vi "Furnace_VI.vi"() -> ()   [LabVIEW 2014]
uses:
  <vilib>/rvi/Emulation/niFpgaGetClockAttributes.vi
  <vilib>/rvi/Emulation/niFpgaSctlEmulationGetInTimedLoop.vi
  <vilib>/rvi/Emulation/niFpgaEmulationReportErrorSimple.vi
  <vilib>/rvi/Emulation/niFpgaCriticalErrorInLSC.vi
panel:
  out "appended array":u8[](array[numeric])
  in  "Command":i16
  in  "Ramp rate,SP&CRC":u8[](array[numeric])=[66, 0, 0, 0, 132, 246]
  in  "Furnace Array Out":u8[](array[numeric])=[65, 48, 48, 48, 48, 48, 13, 68, 48, 48, 48, 48]
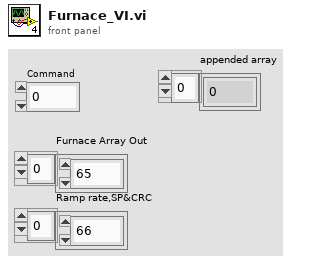
[diagram p1: front panel]
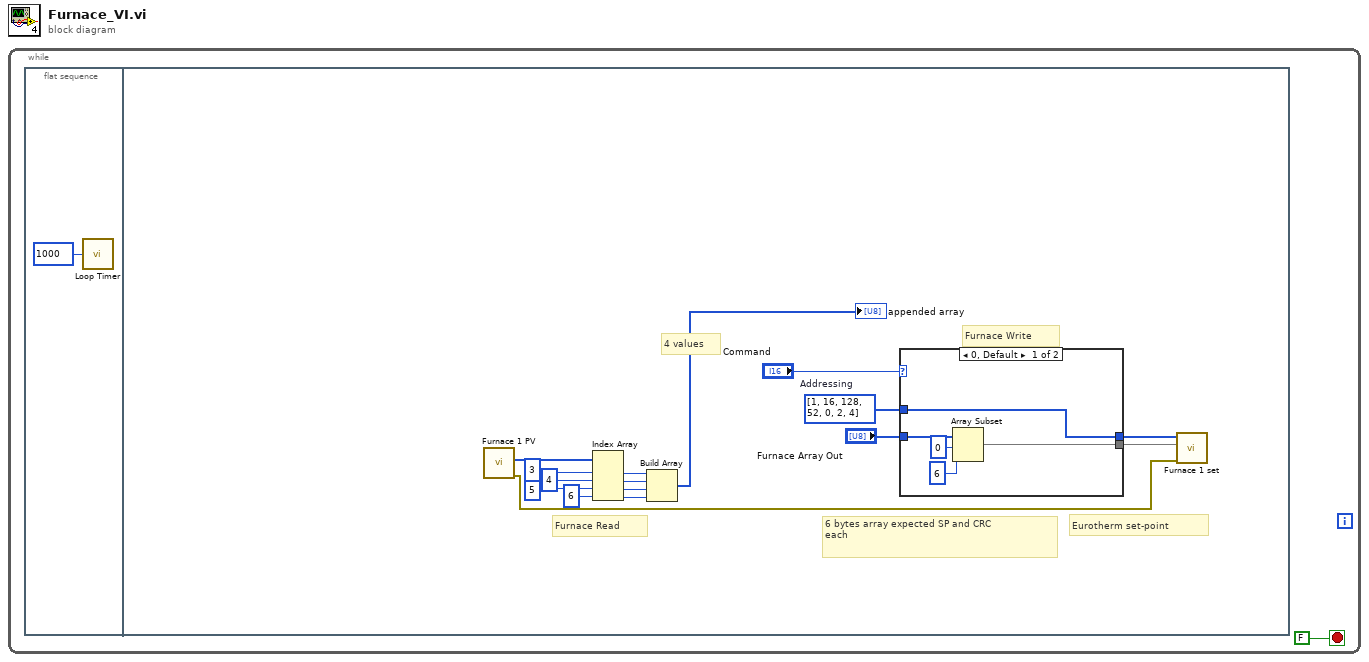
[diagram p0: block diagram]
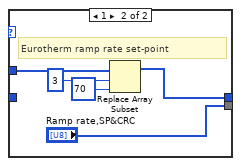
[diagram p2: hidden frame]
diagram:
  n1 = while {
    stop <- FALSE ("stop") stop-if-true
    n2 = flat-sequence {
      frame #0 {
        n3 = call "Loop Timer"("Count(mSec)"=u32 1000) -> ()  [unwired: 1 out]
      }
      frame #1 {
        w5 = u8[] [1, 16, 128, 52, 0, 2, 4]  # Addressing
        # "Furnace Write"
        # "Furnace Read"
        # "4 values"
        # "6 bytes array expected SP and CRC\neach"
        # "Eurotherm set-point"
        n4 = call "Furnace 1 PV.vi"() -> ("error out"=w6:errorcluster, "Array"=w17:u8[])  [unwired: 10 in]
        n5 = Index Array(array=w17, index #1=3, index #2=4, index #3=5, index #4=6 ("index")) -> (element #1=w9:u8, element #2=w10:u8, element #3=w11:u8, element #4=w12:u8)
        n6 = Build Array(w9, w10, w11, w12) -> (→"appended array":u8[])
        n7 = case shown="0, Default" "Command" {
          tunnel: [w20 w26] -> w7
          tunnel: "Furnace Array Out" -> [w21 _]
          tunnel: [w19 "Ramp rate,SP&CRC"] -> w18
          tunnel: w5 -> [w20 w27]
          frame 0, Default {
            n8 = Array Subset(array=w21, index=0, length=6) -> (w19:u8[])
          }
          frame 1 {
            # "Eurotherm ramp rate set-point"
            n9 = Replace Array Subset(array=w27, new element=u8 70 ("new element/subarray"), index=3) -> (w26:u8[])
          }
        }
        n10 = call "Furnace 1 set.vi"("error in"=w6, "SP&CRC"=w18, "Addressing"=w7) -> ()  [unwired: 8 in, 1 out]
      }
    }
  }
